vi "SimpleFrameParser.vi"(6 "SimpleFrameParserState":T1, 9 "data":u8) -> (0 "SimpleFrameParserStateOut":T1, 1 "frameComplete":bool, 3 "frame_data":u8[](array[numeric]))   [LabVIEW 2017]
uses:
  SimpleFrameParserState.ctl
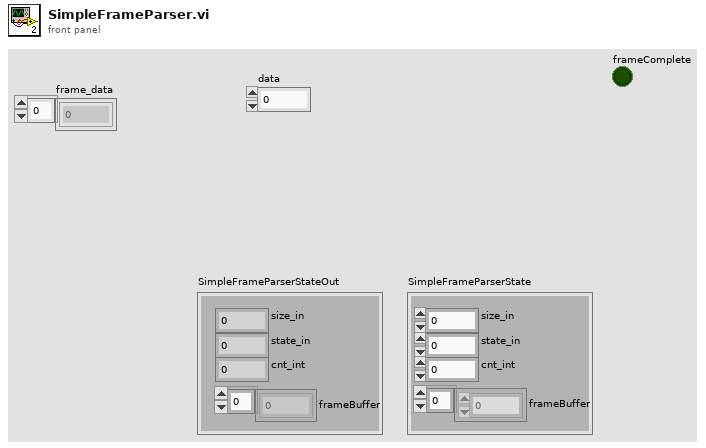
[diagram p1: front panel]
types:
  T1 = typedef "SimpleFrameParserState.ctl" = cluster{"state_in":i32, "cnt_int":i32, "size_in":i32, "frameBuffer":u8[]}
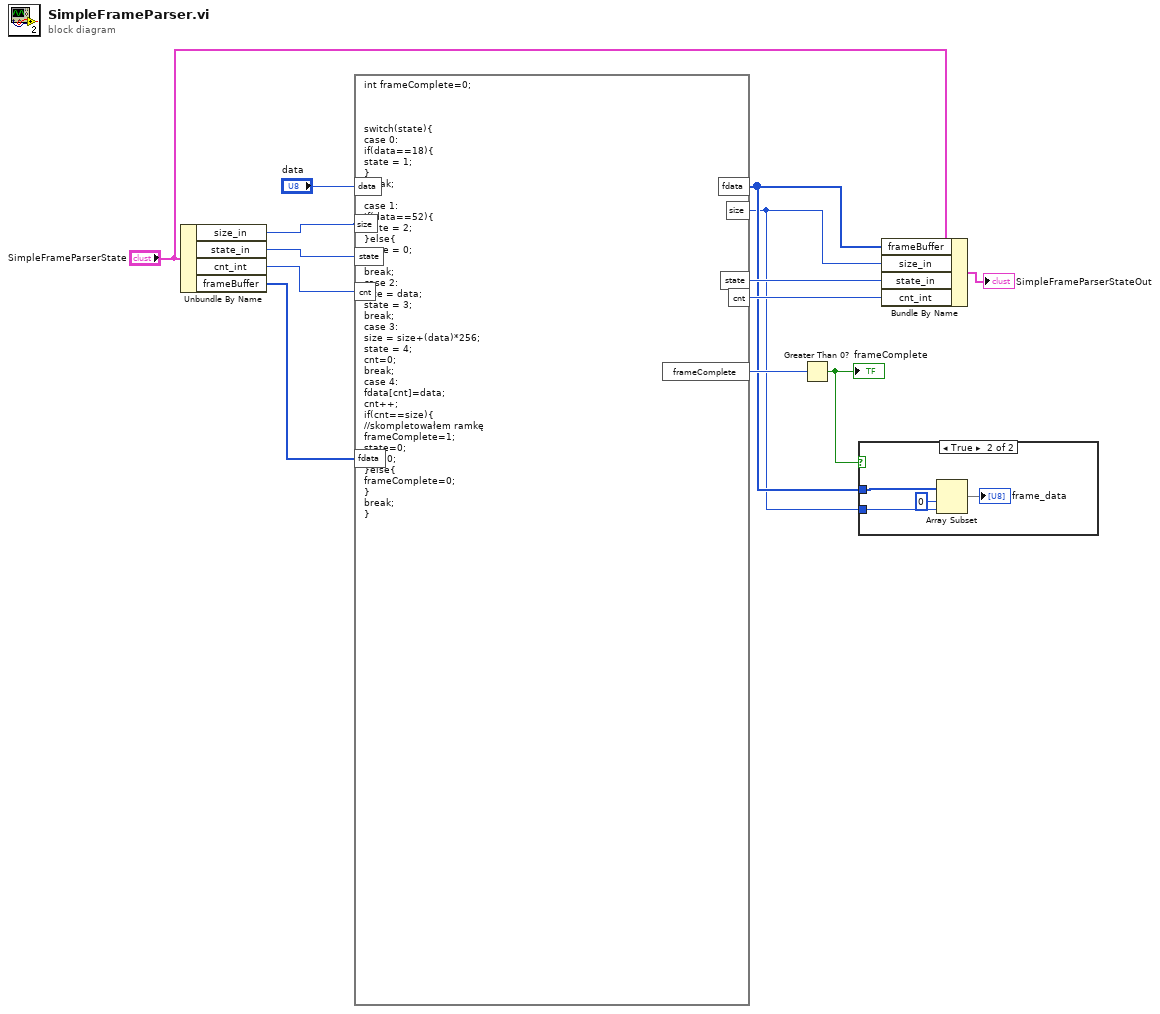
[diagram p0: block diagram]
diagram:
  n1 = Unbundle By Name("SimpleFrameParserState") -> ("size_in"=w12:i32, "state_in"=w11:i32, "cnt_int"=w10:i32, "frameBuffer"=w4:u8[])
  n2 = formula code="int frameComplete=0;\n\n\n\nswitch(state){\ncase 0:\nif(data==18){\nstate = 1;\n}\nbreak;\n\ncase 1:\nif(data==52){\nstate = 2;\n}else{\nstate = 0;\n}\nbreak;\ncase 2:\nsize = data;\nstate = 3;\nbreak;  \ncase 3:\nsize = size+(data)*256;\nstate = 4;\ncnt=0;\nbreak;\ncase 4:\nfdata[cnt]=data;\ncnt++;\nif(cnt==size){\n//skompletowałem ramkę\nframeComplete=1;\nstate=0;\ncnt=0;\n}else{\nframeComplete=0;\n}\nbreak;\n}"("data"="data", "size"=w12, "state"=w11, "fdata"=w4, "cnt"=w10) -> ("fdata"=w2:u8[], "size"=w1:i32, "state"=w7:i32, "cnt"=w6:i32, "frameComplete"=w5:i32)
  n3 = Greater Than 0?(x=w5) -> (x > 0?=w3:bool)
  "frameComplete" <- w3
  n4 = case shown="True" w3 {
    tunnel: w2 -> [_ w17]
    tunnel: w1 -> [_ w16]
    frame False {
    }
    frame True {
      n5 = Array Subset(array=w17, index=0, length=w16) -> (→"frame_data":u8[])
    }
  }
  n6 = Bundle By Name(cluster="SimpleFrameParserState", "frameBuffer"=w2, "size_in"=w1, "state_in"=w7, "cnt_int"=w6) -> (→"SimpleFrameParserStateOut":T1)
